vi "Raise Event.vi"(8 "error in (no error)":errorcluster, 10 "EventData":refnum<class "EventData.lvclass">, 11 "EventManager in":refnum<class "EventManager.lvclass">) -> (0 "error out":errorcluster, 3 "EventManager out":refnum<class "EventManager.lvclass">)   [LabVIEW 2021, in "EventManagerLibrary.lvlib" / "EventManager.lvclass"]
doc: "Raises all the events the Event Manager contains that are typed with the object on the EventData wire. It also removes any invalid Events that it finds.\n\nThis vi runs normally even if an error occurred before this vi."
uses:
  EventManager.lvclass
  EventDataObject/EventData.lvclass
  EventManager.lvclass/EventManager.ctl
  EventBag/EventBag.lvclass
  EventObject/Event.lvclass
  EventToken/EventToken.lvclass
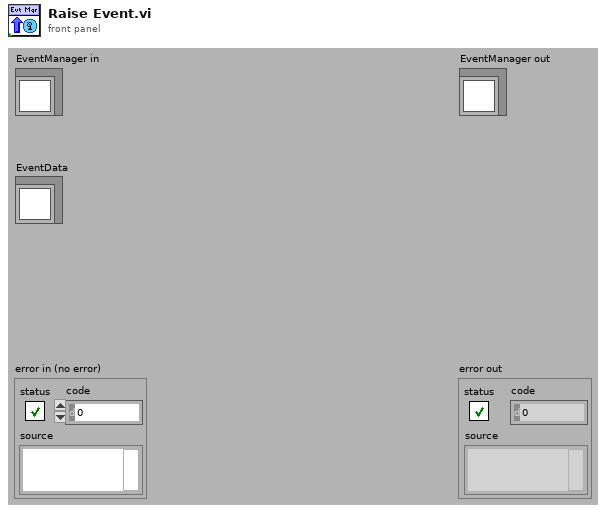
[diagram p1: front panel]
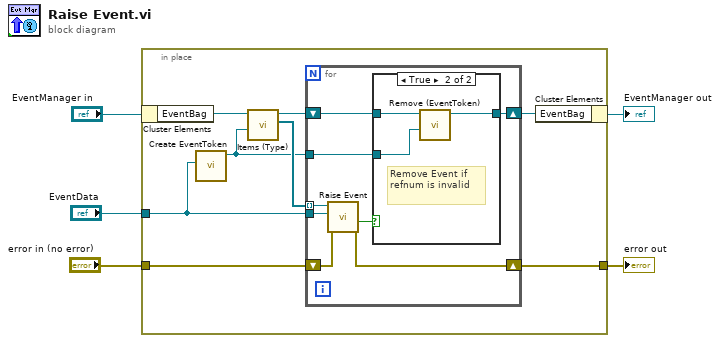
[diagram p0: block diagram]
diagram:
  n1 = in-place {
    in-place-border: "EventData" -> [w7]
    in-place-border: "error in (no error)" -> [w11]
    in-place-border: [w10] -> w1
    n2 = in-place-cluster #1("EventManager in") -> ("EventBag"=w13:refnum<class "EventBag.lvclass">)
    n3 = call "Create EventToken.vi"("EventData Class"=w7) -> ("EventToken out"=w6:refnum<class "EventToken.lvclass">)  [unwired: 2 in, 8 out]
    n4 = call-dynamic "Items (Type).vi"("EventToken"=w6, "EventBag in"=w13) -> ("Events"=w12:refnum<class "Event.lvclass">[], "EventBag out"=w9:refnum<class "EventBag.lvclass">)  [unwired: 1 in, 7 out]
    n5 = for {
      tunnel: w12 -> [w21] mode=indexing
      tunnel: w7 -> [w20]
      shift-right: [w18] -> w10
      shift-left: w11 -> [w19]
      shift-right: [w15] -> w8
      shift-left: w9 -> [w16]
      tunnel: w6 -> [w14]
      n6 = call "Raise Event.vi"("error in (no error)"=w19, "EventDataObj"=w20, "Event in"=w21) -> ("error out"=w18:errorcluster, "InvalidEventRef?"=w17:bool)  [unwired: 7 out]
      n7 = case shown="True" w17 {
        tunnel: w16 -> [w22 w25]
        tunnel: [w22 w24] -> w15
        tunnel: w14 -> [_ w23]
        frame False {
        }
        frame True {
          # "Remove Event if refnum is invalid"
          n8 = call-dynamic "Remove (EventToken).vi"("EventToken"=w23, "EventBag in"=w25) -> ("EventBag out"=w24:refnum<class "EventBag.lvclass">)  [unwired: 1 in, 8 out]
        }
      }
    }
    n9 = in-place-cluster #1("EventBag"=w8) -> (→"EventManager out":refnum<class "EventManager.lvclass">)
  }
  "error out" <- w1
